vi "Format Step String.vi"(8 "Initial string (default: \"Step\")":string="Step", 10 "Description":string, 11 "Step Number":i32) -> (3 "Step String out":string)   [LabVIEW 2020, in "Output Sequencer.lvlib" / "Settings UI.lvclass"]
uses:
  Settings UI.lvclass
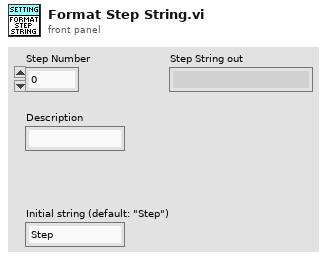
[diagram p1: front panel]
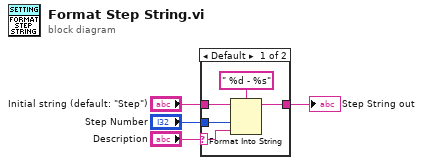
[diagram p0: block diagram]
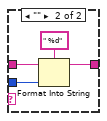
[diagram p2: hidden frame]
diagram:
  n1 = case shown="Default" "Description" {
    selector: "Description" -> [w6 _]
    tunnel: "Step Number" -> [w7 w13]
    tunnel: [w8 w12] -> w2
    tunnel: "Initial string (default: \"Step\")" -> [w5 w10]
    frame Default {
      n2 = Format Into String(format string=" %d - %s", initial string=w5, w7, w6) -> (resulting string=w8:string)  [unwired: 1 in, 1 out]
    }
    frame "" {
      n3 = Format Into String(format string=" %d", initial string=w10, w13) -> (resulting string=w12:string)  [unwired: 1 in, 1 out]
    }
  }
  "Step String out" <- w2
